vi "AddArgument.vi"(8 "error in (no error)":errorcluster, 10 "ArgumentConfig":refnum<class "ArgumentConfig.lvclass">, 11 "ArgumentParser in":refnum<class "ArgumentParser.lvclass">) -> (0 "error out":errorcluster, 3 "ArgumentParser out":refnum<class "ArgumentParser.lvclass">)   [LabVIEW 2022 SP3, in "ArgumentParser.lvlib" / "ArgumentParser.lvclass"]
uses:
  ArgumentParser.lvclass
  ArgumentConfig/ArgumentConfig.lvclass
  ArgumentConfig/ArgumentConfig.lvclass/ArgumentConfig.ctl
  ArgumentParser.lvclass/ArgumentParser.ctl
  ArgumentConfig/Read NameOrFlags.vi
  ArgumentConfig/Read Action.vi
  ArgumentConfig/Read NumberOfArguments.vi
  ArgumentConfig/Read Constant.vi
  ArgumentConfig/Read Default.vi
  ArgumentConfig/Read Choices.vi
  ArgumentConfig/Read Required.vi
  ArgumentConfig/Read Help.vi
  ArgumentConfig/Read Metavar.vi
  ArgumentConfig/Read Destination.vi
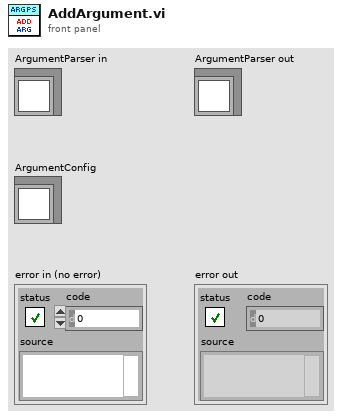
[diagram p1: front panel]
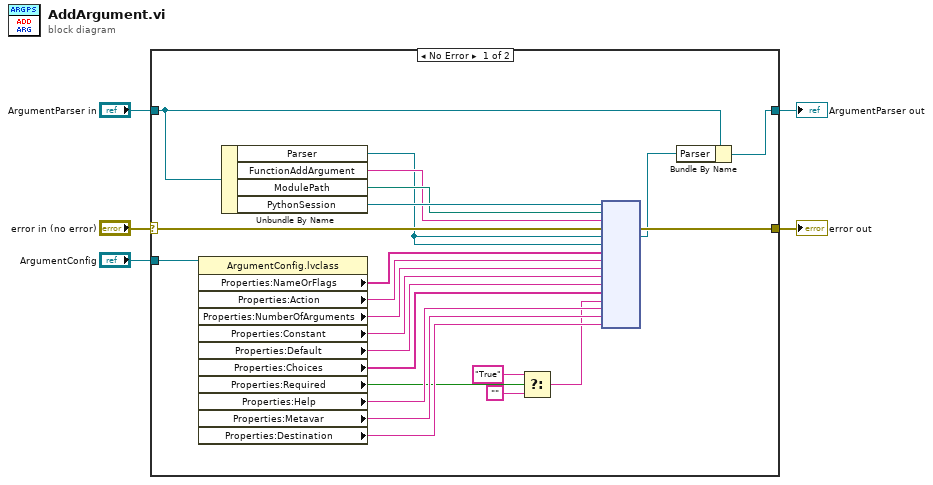
[diagram p0: block diagram]
diagram:
  n1 = case shown="No Error" "error in (no error)" {
    selector: "error in (no error)" -> [w28 w30]
    tunnel: [w27 w30] -> w4
    tunnel: [w11 w29] -> w2
    tunnel: "ArgumentParser in" -> [w10 w29]
    tunnel: "ArgumentConfig" -> [w23 _]
    frame No Error {
      n2 = property class="ArgumentConfig.lvclass"(reference=w23) -> ("Properties:NameOrFlags"=w22:string[], "Properties:Action"=w21:string, "Properties:NumberOfArguments"=w20:string, "Properties:Constant"=w19:string, "Properties:Default"=w18:string, "Properties:Choices"=w17:string[], "Properties:Required"=w9:bool, "Properties:Help"=w16:string, "Properties:Metavar"=w15:string, "Properties:Destination"=w14:string)  [unwired: 1 in, 2 out]
      n3 = Unbundle By Name(w10) -> ("Parser"=w13:refnum<k38>, "FunctionAddArgument"=w24:string, "ModulePath"=w25:path, "PythonSession"=w26:refnum<k35>)
      n4 = Select(t="True", s=w9, f="") -> (s? t:f=w8:string)
      n5 = node(w26, w25, w24, w28, w13, w13, w22, w21, w20, w19, w18, w17, w8, w16, w15, w14) -> (w27:errorcluster, w12:refnum<k38>)  [unwired: 11 in, 3 out]
      n6 = Bundle By Name(cluster=w10, "Parser"=w12) -> (w11:refnum<class "ArgumentParser.lvclass">)
    }
    frame Error {
    }
  }
  "error out" <- w4
  "ArgumentParser out" <- w2
